vi "Mixtime.vi"(10 "Mixtime(ms)":u32=5000) -> ()   [LabVIEW 2019]
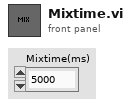
[diagram p1: front panel]
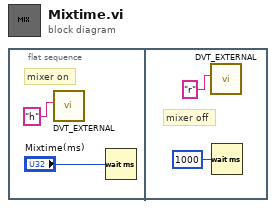
[diagram p0: block diagram]
diagram:
  n1 = flat-sequence {
    frame #0 {
      # "mixer on"
      n2 = call "DVT_EXTERNAL.vi"("write buffer"="h") -> ()  [unwired: 3 in, 3 out]
      n3 = Wait (ms)(milliseconds to wait="Mixtime(ms)") -> ()  [unwired: 1 out]
    }
    frame #1 {
      # "mixer off"
      n4 = call "DVT_EXTERNAL.vi"("write buffer"="r") -> ()  [unwired: 3 in, 3 out]
      n5 = Wait (ms)(milliseconds to wait=u32 1000) -> ()  [unwired: 1 out]
    }
  }
